vi "MC.SetWavelength.vi"(8 "error in (no error)":errorcluster, 10 "Wavelength, nm":dbl=620.0, 11 "MC.DangwooOptron":refnum<class "MC.DangwooOptron.lvclass">) -> (0 "error out":errorcluster, 3 "MC.DangwooOptron out":refnum<class "MC.DangwooOptron.lvclass">)   [LabVIEW 2017, in "MC.DangwooOptron.lvclass"]
doc: "---------------------------------------------------------------\nJKI State Machine Objects™\nhttp://jki.net/state-machine-objects/\nCopyright (C) 2005-2015, JKI <info@jki.net>\nALL RIGHTS RESERVEDJKI State Machine Objects (SMO) 1.0.0.5\nJKI - JKI\nCopyright (c) 2016, JKI"
uses:
  MC.DangwooOptron.lvclass
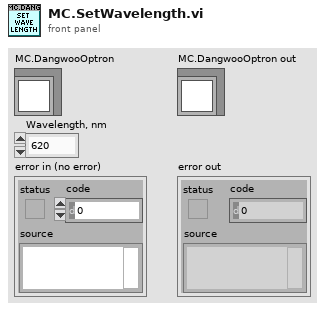
[diagram p1: front panel]
types:
  T1 = typedef "MC.DangwooOptron.lvclass/Resource--Cluster.ctl" = cluster{"VISA resource":refnum<visa-resource-name>}
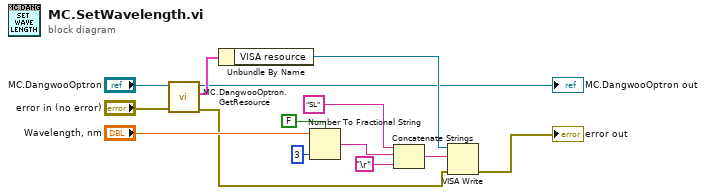
[diagram p0: block diagram]
diagram:
  n1 = call "MC.DangwooOptron.GetResource.vi"("error in (no error)"="error in (no error)", "MC.DangwooOptron"="MC.DangwooOptron") -> ("error out"=w4:errorcluster, "Resource"=w6:T1, "MC.DangwooOptron out"=→"MC.DangwooOptron out":refnum<class "MC.DangwooOptron.lvclass">)  [unwired: 7 in]
  n2 = Unbundle By Name(w6) -> ("VISA resource"=w5:refnum<visa-resource-name>)
  n3 = Number To Fractional String(use system decimal point (T)=FALSE, number="Wavelength, nm", precision (6)=3) -> (F-format string=w10:string)  [unwired: 1 in]
  n4 = Concatenate Strings("SL" ("SL"), w10, "\r") -> (w12:string)
  n5 = VISA Write(VISA resource name=w5, write buffer=w12, error in (no error)=w4) -> (error out=→"error out":errorcluster)  [unwired: 2 out]
